vi "obtain_latest_instance.vi"(7 "quick, but maybe outdated?":bool=TRUE, 8 "error in (no error)":errorcluster) -> (0 "error out":errorcluster, 3 "GenericDAQ out":refnum<class "GenericDAQ.lvclass">)   [LabVIEW 2010, in "GenericDAQ.lvclass"]
uses:
  GenericDAQ.lvclass
  common/classes/ErrorController/ErrorController/class_data.vi
  class_data.vi
  common/classes/ErrorController/ErrorController/ErrorController.lvclass
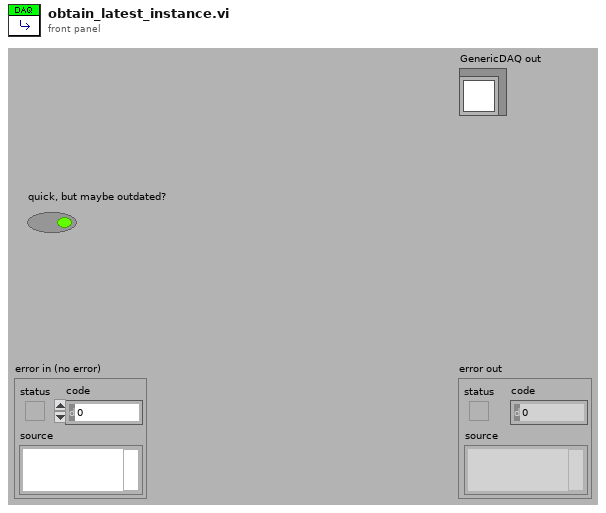
[diagram p1: front panel]
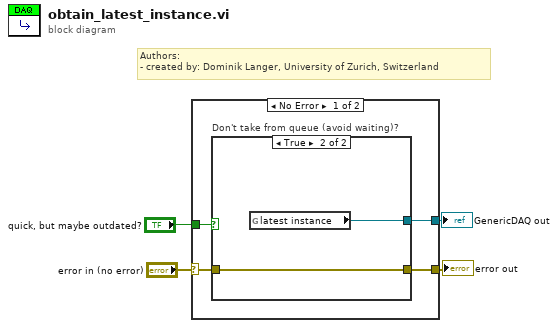
[diagram p0: block diagram]
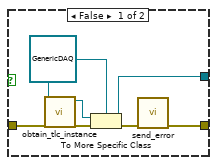
[diagram p2: hidden frame]
diagram:
  # "Authors: \n- created by: Dominik Langer, University of Zurich, Switzerland"
  n1 = case shown="No Error" "error in (no error)" {
    selector: "error in (no error)" -> [w6 w18]
    tunnel: [w8 w18] -> w3
    tunnel: [w7 _] -> w2
    tunnel: "quick, but maybe outdated?" -> [w5 _]
    frame No Error {
      n2 = case "Don't take from queue (avoid waiting)?" shown="True" w5 {
        tunnel: [w13 w16] -> w8
        tunnel: [w15 w17] -> w7
        tunnel: w6 -> [w9 w16]
        frame False {
          w12 = refnum<class "GenericDAQ.lvclass"> refnum ("GenericDAQ.lvclass")
          n3 = call-dynamic "obtain_tlc_instance.vi"("error in (no error)"=w9, "GenericToplevelComponent in"=w12) -> ("error out"=w10:errorcluster, "GenericToplevelComponent out"=w11:refnum<class "GenericToplevelComponent.lvclass">)  [unwired: 8 in]
          n4 = To More Specific Class(target class=w12, reference=w11, error in=w10) -> (specific class reference=w15:refnum<class "GenericDAQ.lvclass">, error out=w14:errorcluster)
          n5 = call "send_error.vi"("error in (no error)"=w14) -> ("error out"=w13:errorcluster)  [unwired: 10 in]
        }
        frame True {
          n6 = global read "class_data.vi" "latest instance"() -> (w17:refnum<class "GenericDAQ.lvclass">)
        }
      }
    }
    frame Error {
    }
  }
  "error out" <- w3
  "GenericDAQ out" <- w2
